vi "DDC (Multi-Channel, IQ Power Trigger).vi"(0 "data in":T2[](array[typedef])=[{"I"=0.0, "Q"=0.0, "overflow"=FALSE}, {"I"=0.0, "Q"=0.0, "overflow"=FALSE}], 1 "reset":bool, 5 "start trigger":bool, 7 "power level trigger configuration":T1 {"trig level" format="%#.48g"}, 9 "enabled":bool[](array[boolean])=[FALSE, FALSE], 11 "DDC Parameters":T3[](array[typedef])=[{"output sample rate"=0.0, "delay"=0.0, "frequency shift"=0.0, "impairments"={"inline gain I"=0.0, "inline gain Q"=0.0, "cross gain I"=0.0, "cross gain Q"=0.0, "pre-gain offset I"=0.0, "pre-gain offset Q"=0.0, "post-gain offset I"=0.0, "post-gain offset Q"=0.0}, "phase"=0.0}, {"output sample rate"=0.0, "delay"=0.0, "frequency shift"=0.0, "impairments"={"inline gain I"=0.0, "inline gain Q"=0.0, "cross gain I"=0.0, "cross gain Q"=0.0, "pre-gain offset I"=0.0, "pre-gain offset Q"=0.0, "post-gain offset I"=0.0, "post-gain offset Q"=0.0}, "phase"=0.0}] {"frequency shift" format="%#.48g"}, 13 "ready for trigger":bool=TRUE) -> (4 "data out":u32[](array[numeric]), 6 "number of overflows":u64[](array[numeric]), 8 "power level triggers":bool[](array[boolean]), 10 "output valid":bool, 14 "dsp reset done":bool)   [LabVIEW 2023]
doc: "Controls whether or not data is written to the DMA FIFO for the acquisition stream. If burst size is 0, this will be a continuous stream, started when the start trigger is asserted. If burst size is greater than zero, acquisition will be in bursts of the designated size, initiated each time the internal state machine is idle and a start trigger is received.\n\nThis VI also keeps track of whether or not an overflow occurred in the acquisition stream and counts the number of overflows that have occurred for debugging information.\n\nThe internal state machine returns the number of samples processed since the most recent acquisition began and the current state machine state."
uses:
  <instrlib>/_niInstr/DSP/v1/Shared/Public/IQ Data.ctl
  <instrlib>/_niInstr/DSP/v1/Shared/Public/IQ Impairments.ctl
  <instrlib>/niUSRP/Reference FPGA/SubVIs/DDC Parameters.ctl
  <instrlib>/_niInstr/DSP/v1/Shared/Public/IQ Power Level Configuration - 36 bit.ctl
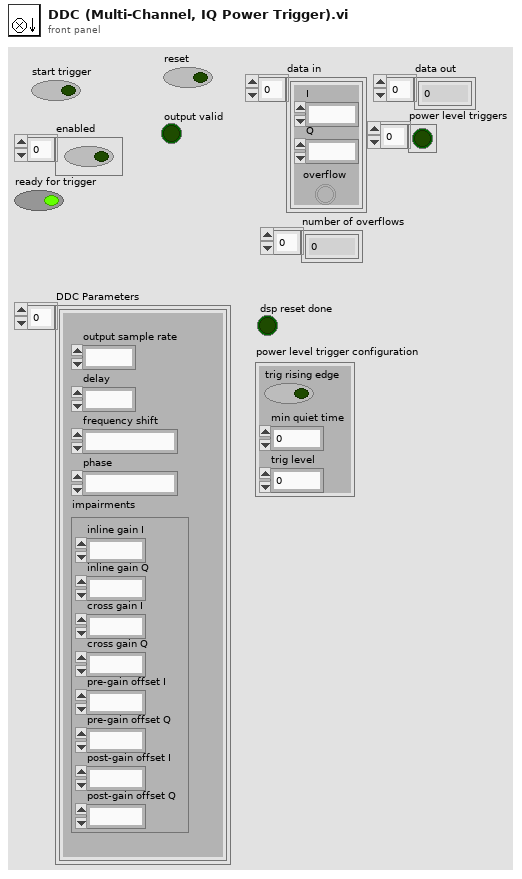
[diagram p1: front panel]
types:
  T1 = typedef "niInstr DSP v1 Shared.lvlib/IQ Power Level Configuration - 36 bit.ctl" = cluster{"trig rising edge":bool, "min quiet time":u32, "trig level":fxp<+,36,2>}
  T2 = typedef "niInstr DSP v1 Shared.lvlib/IQ Data.ctl" = cluster{"I":fxp<+/-,18,1>, "Q":fxp<+/-,18,1>, "overflow":bool}
  T3 = typedef "DDC Parameters.ctl" = cluster{"output sample rate":fxp<+,48,1>, "delay":fxp<+/-,16,0>, "frequency shift":fxp<+/-,48,0>, "impairments":T4, "phase":fxp<+/-,21,0>}
  T4 = typedef "niInstr DSP v1 Shared.lvlib/IQ Impairments.ctl" = cluster{"inline gain I":fxp<+/-,18,1>, "inline gain Q":fxp<+/-,18,1>, "cross gain I":fxp<+/-,18,1>, "cross gain Q":fxp<+/-,18,1>, "pre-gain offset I":fxp<+/-,18,1>, "pre-gain offset Q":fxp<+/-,18,1>, "post-gain offset I":fxp<+/-,18,1>, "post-gain offset Q":fxp<+/-,18,1>}
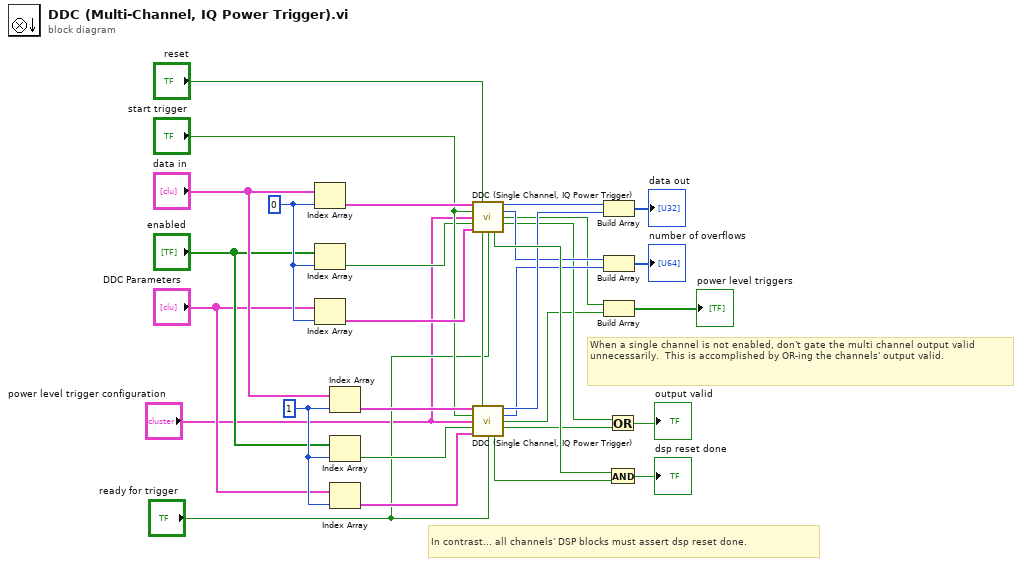
[diagram p0: block diagram]
diagram:
  w27 = 1 ("index")
  w28 = 0 ("index")
  # "When a single channel is not enabled, don't gate the multi channel output valid unnecessarily.  This is accomplished by OR-ing the channels' output valid."
  # "In contrast... all channels' DSP blocks must assert dsp reset done."
  n1 = Index Array(array="data in", index=w28) -> (element=w30:T2)
  n2 = Index Array(array="enabled", index=w28) -> (element=w9:bool)
  n3 = Index Array(array="DDC Parameters", index=w28) -> (element=w29:T3)
  n4 = Index Array(array="data in", index=w27) -> (element=w23:T2)
  n5 = Index Array(array="enabled", index=w27) -> (element=w8:bool)
  n6 = Index Array(array="DDC Parameters", index=w27) -> (element=w22:T3)
  n7 = call <instrlib>:"DDC (Single Channel, IQ Power Trigger).vi"("data in"=w30, "reset"="reset", "start trigger"="start trigger", "power level trigger configuration"="power level trigger configuration", "enabled"=w9, "DDC Parameters"=w29, "ready for trigger"="ready for trigger") -> ("data out"=w15:u32, "number of overflows"=w12:u64, "power level trigger"=w3:bool, "output valid"=w6:bool, "dsp reset done"=w19:bool)  [unwired: 4 in]
  n8 = call <instrlib>:"DDC (Single Channel, IQ Power Trigger).vi"("data in"=w23, "reset"="reset", "start trigger"="start trigger", "power level trigger configuration"="power level trigger configuration", "enabled"=w8, "DDC Parameters"=w22, "ready for trigger"="ready for trigger") -> ("data out"=w13:u32, "number of overflows"=w11:u64, "power level trigger"=w2:bool, "output valid"=w7:bool, "dsp reset done"=w18:bool)  [unwired: 4 in]
  n9 = Build Array(w15, w13) -> (→"data out":u32[])
  n10 = Build Array(w12, w11) -> (→"number of overflows":u64[])
  n11 = Build Array(w3, w2) -> (→"power level triggers":bool[])
  n12 = Or(x=w6, y=w7) -> (x .or. y?=→"output valid":bool)
  n13 = And(x=w19, y=w18) -> (x .and. y?=→"dsp reset done":bool)
